vi "Shoot.vi"(0 "Shoot during x ms":dbl, 1 "Arduino Serial Port":refnum<visa-resource-name>, 2 "error in (no error)":errorcluster caption="entrée d'erreur (pas d'erreur)") -> (3 "Arduino Serial out":refnum<visa-resource-name>, 4 "Message":string, 5 "Shot Unitil":dbl, 6 "error out":errorcluster caption="sortie d'erreur")   [LabVIEW 2014, in "ShootingStar.lvlib"]
uses:
  ShootingStar.lvlib
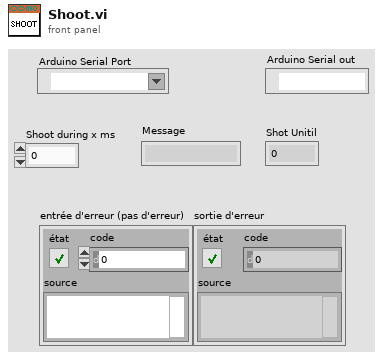
[diagram p1: front panel]
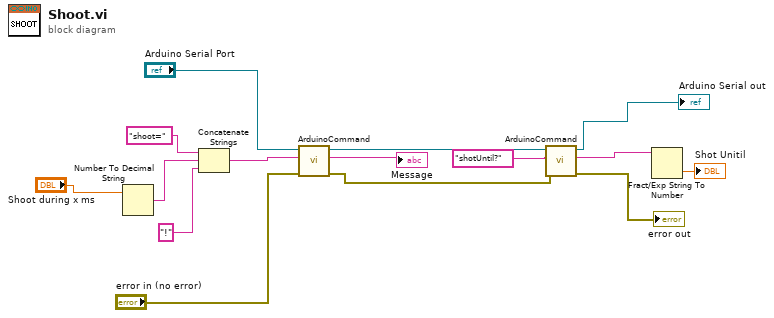
[diagram p0: block diagram]
diagram:
  n1 = Number To Decimal String(number="Shoot during x ms") -> (decimal integer string=w12:string)  [unwired: 1 in]
  n2 = Concatenate Strings("shoot=" ("buffer à écrire"), w12, "!") -> (w9:string)
  n3 = call "ArduinoCommand.vi"("entrée d'erreur (pas d'erreur)"="error in (no error)", "buffer à écrire"=w9, "Refnum VISA en entrée"="Arduino Serial Port") -> ("sortie d'erreur"=w6:errorcluster, "read buffer"=→"Message":string, "Refnum VISA en sortie"=w7:refnum<visa-resource-name>)  [unwired: 6 in]
  n4 = call "ArduinoCommand.vi"("entrée d'erreur (pas d'erreur)"=w6, "buffer à écrire"="shotUntil?" ("write buffer"), "Refnum VISA en entrée"=w7) -> ("sortie d'erreur"=→"error out":errorcluster, "read buffer"=w3:string, "Refnum VISA en sortie"=→"Arduino Serial out":refnum<visa-resource-name>)  [unwired: 6 in]
  n5 = Fract/Exp String To Number(string=w3) -> (number=→"Shot Unitil":dbl)  [unwired: 3 in, 1 out]
